vi "PBL2.vi"() -> ()   [LabVIEW 2017]
uses:
  C:/Users/mjoha/Documents/School/ELIC328/LabViewProject/FanCtrl/LabView Fan Controller.dll
  LabView Fan Controller.dll
panel:
  out "?":bool
  in  "COM Port":string
  in  "stop":bool
  in  "Temperature Settings":T1
  in  "?":enum32{"Output", "Settings", "Error Output"}(tab)
  out "Tempurate\nZone 2":dbl
  out "Tempurate\nZone 1":dbl
  out "Waveform Chart":T2(graph)
  in  "Zone 2":T3
  in  "Zone 1":T3
  out "error out":errorcluster
  # "Zone 1"
  # "Min"
  # "Max"
  # "Zone 2"
  # "Max"
  # "Min"
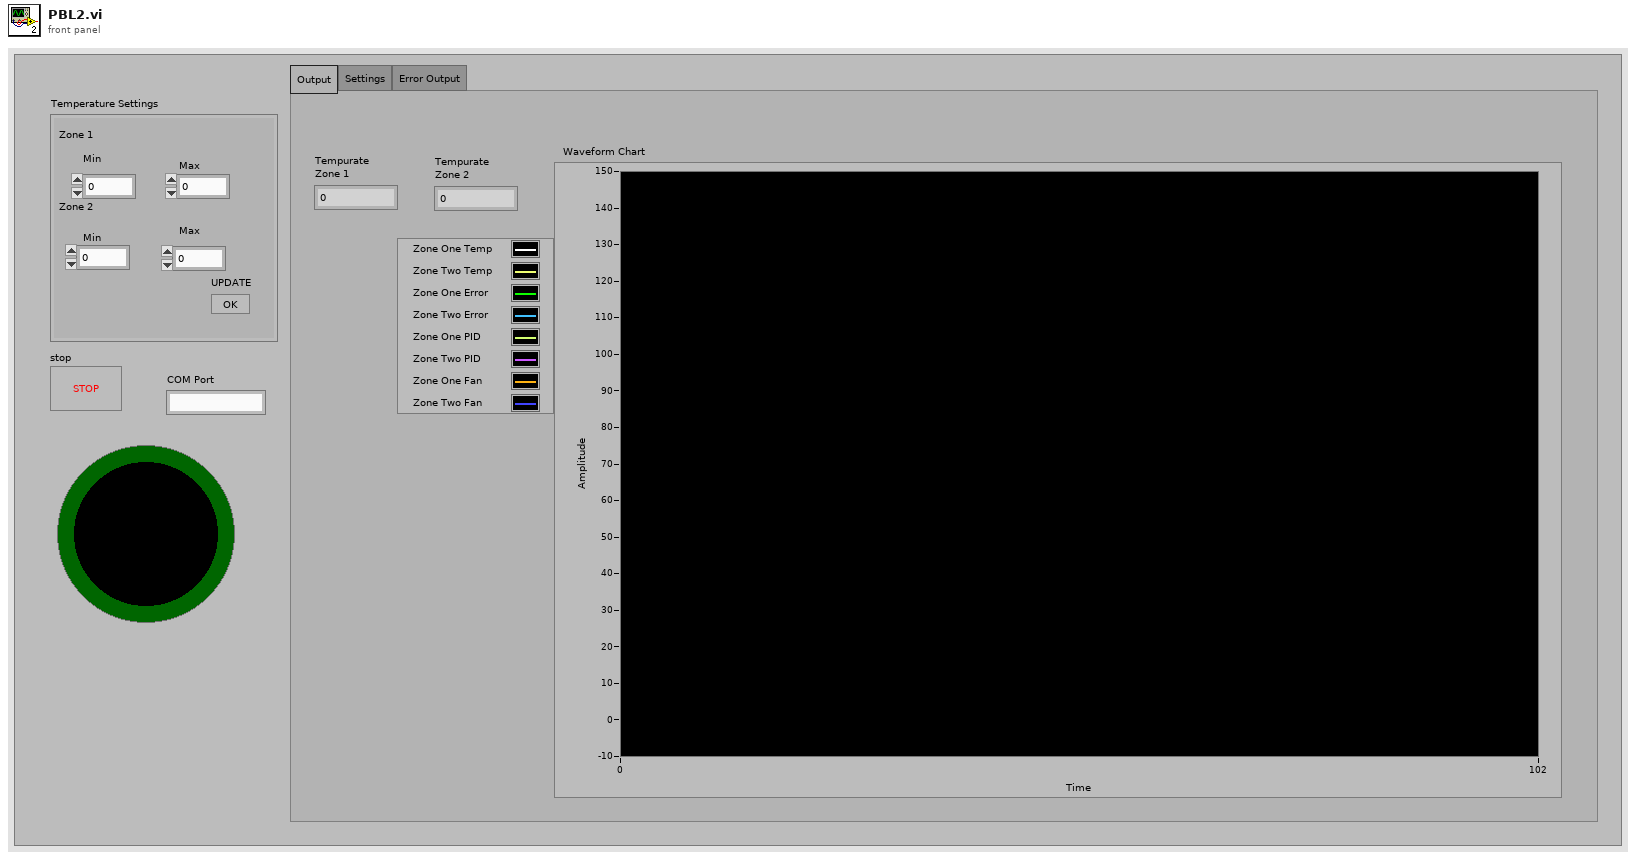
[diagram p1: front panel]
types:
  T1 = cluster{"Zone One Min Temp":dbl, "Zone One Max Temp":dbl, "Zone Two Min Temp":dbl, "Zone Two Max Temp":dbl, "UPDATE":bool}
  T2 = cluster{"ZoneTwoTemperature":dbl, "ZoneOneTemperature":dbl, "ZoneOneError":dbl, "ZoneTwoError":dbl, "ZoneOnePidRate":dbl, "ZoneTwoPidRate":dbl, "ZoneOneFanPwm":i32, "ZoneTwoFanPwm":i32}
  T3 = cluster{"KI":dbl, "KP":dbl, "KD":dbl, "Temp Samp":dbl, "Pid Samp":dbl}
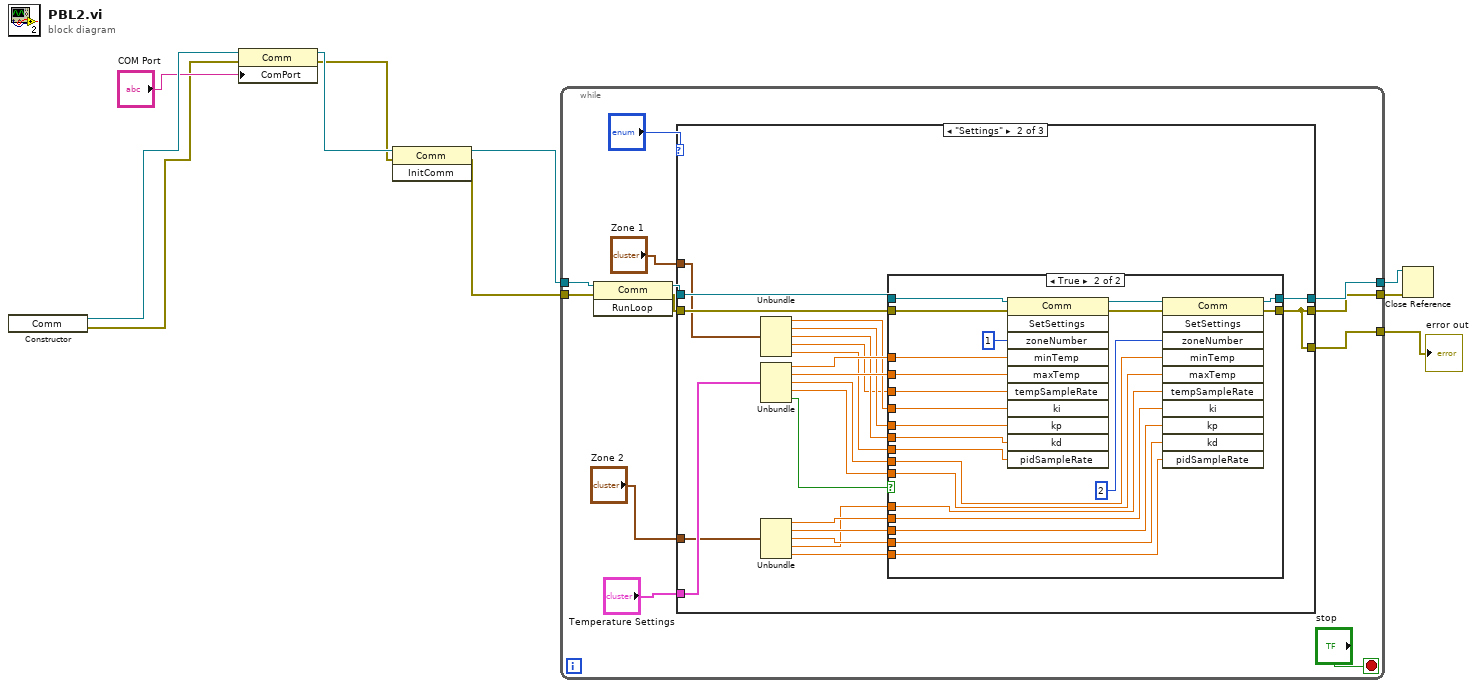
[diagram p0: block diagram]
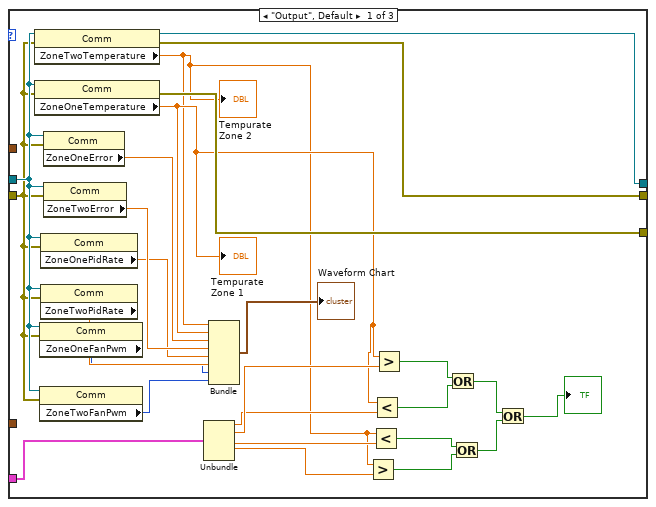
[diagram p2: hidden frame]
diagram:
  n1 = constructor class="Comm"() -> (reference out=w6:refnum<k24>, error out=w4:errorcluster)  [unwired: 3 in, 1 out]
  n2 = property class="Comm"(reference=w6, error in=w4, "ComPort"="COM Port") -> (reference out=w3:refnum<k24>, error out=w2:errorcluster)
  n3 = invoke class="Comm" method="InitComm"(reference=w3, error in=w2) -> (reference out=w8:refnum<k24>, error out=w7:errorcluster)  [unwired: 1 in, 1 out]
  n4 = while {
    tunnel: w8 -> [w19]
    tunnel: w7 -> [w18]
    tunnel: [w21] -> w10
    tunnel: [w20] -> w9
    tunnel: [w11] -> w1
    stop <- "stop" stop-if-true
    n5 = invoke class="Comm" method="RunLoop"(reference=w19, error in=w18) -> (reference out=w17:refnum<k24>, error out=w16:errorcluster)  [unwired: 1 in, 1 out]
    n6 = case shown="\"Settings\"" "?" {
      tunnel: w17 -> [w46 w69 w94]
      tunnel: w16 -> [w45 w68 w93]
      tunnel: [w48 w59 w94] -> w21
      tunnel: [w47 w50 w93] -> w20
      tunnel: "Temperature Settings" -> [w36 w70 _]
      tunnel: "Zone 1" -> [_ w65 _]
      tunnel: "Zone 2" -> [_ w58 _]
      tunnel: [w37 w50 w93] -> w11
      frame "Output", Default {
        n7 = property class="Comm"(reference=w46, error in=w45) -> (reference out=w48:refnum<k24>, error out=w47:errorcluster, "ZoneTwoTemperature"=w31:dbl)
        "Tempurate\nZone 2" <- w31
        n8 = property class="Comm"(reference=w46, error in=w45) -> (error out=w37:errorcluster, "ZoneOneTemperature"=w34:dbl)  [unwired: 1 out]
        "Tempurate\nZone 1" <- w34
        n9 = property class="Comm"(reference=w46, error in=w45) -> ("ZoneOneFanPwm"=w40:i32)  [unwired: 2 out]
        n10 = property class="Comm"(reference=w46, error in=w45) -> ("ZoneTwoFanPwm"=w39:i32)  [unwired: 2 out]
        n11 = property class="Comm"(reference=w46, error in=w45) -> ("ZoneOnePidRate"=w42:dbl)  [unwired: 2 out]
        n12 = property class="Comm"(reference=w46, error in=w45) -> ("ZoneTwoPidRate"=w41:dbl)  [unwired: 2 out]
        n13 = property class="Comm"(reference=w46, error in=w45) -> ("ZoneOneError"=w44:dbl)  [unwired: 2 out]
        n14 = property class="Comm"(reference=w46, error in=w45) -> ("ZoneTwoError"=w43:dbl)  [unwired: 2 out]
        n15 = Unbundle(w36) -> ("Zone One Min Temp"=w33:dbl, "Zone One Max Temp"=w35:dbl, "Zone Two Min Temp"=w32:dbl, "Zone Two Max Temp"=w30:dbl)  [unwired: 1 out]
        n16 = Bundle("ZoneTwoTemperature"=w31, "ZoneOneTemperature"=w34, "ZoneOneError"=w44, "ZoneTwoError"=w43, "ZoneOnePidRate"=w42, "ZoneTwoPidRate"=w41, "ZoneOneFanPwm"=w40, "ZoneTwoFanPwm"=w39) -> (→"Waveform Chart":T2)  [unwired: 1 in]
        n17 = Greater?(x=w31, y=w30) -> (0:w26:bool)
        n18 = Less?(x=w31, y=w32) -> (x < y?=w27:bool)
        n19 = Less?(x=w34, y=w33) -> (x < y?=w28:bool)
        n20 = Greater?(x=w34, y=w35) -> (0:w29:bool)
        n21 = Or(x=w29, y=w28) -> (x .or. y?=w25:bool)
        n22 = Or(x=w27, y=w26) -> (x .or. y?=w24:bool)
        n23 = Or(x=w25, y=w24) -> (x .or. y?=→"?":bool)
      }
      frame "Settings" {
        n24 = Unbundle(w65) -> ("KI"=w64:dbl, "KP"=w63:dbl, "KD"=w62:dbl, "Temp Samp"=w61:dbl, "Pid Samp"=w60:dbl)
        n25 = Unbundle(w70) -> ("Zone One Min Temp"=w67:dbl, "Zone One Max Temp"=w66:dbl, "Zone Two Min Temp"=w52:dbl, "Zone Two Max Temp"=w51:dbl, "UPDATE"=w49:bool)
        n26 = Unbundle(w58) -> ("KI"=w57:dbl, "KP"=w56:dbl, "KD"=w55:dbl, "Temp Samp"=w54:dbl, "Pid Samp"=w53:dbl)
        n27 = case shown="True" w49 {
          tunnel: w69 -> [_ w92]
          tunnel: w68 -> [_ w91]
          tunnel: [_ w79] -> w50
          tunnel: w67 -> [_ w89]
          tunnel: w66 -> [_ w88]
          tunnel: w64 -> [_ w87]
          tunnel: w63 -> [_ w86]
          tunnel: w62 -> [_ w85]
          tunnel: w61 -> [_ w84]
          tunnel: w60 -> [_ w83]
          tunnel: [_ w80] -> w59
          tunnel: w57 -> [_ w78]
          tunnel: w56 -> [_ w77]
          tunnel: w55 -> [_ w76]
          tunnel: w54 -> [_ w75]
          tunnel: w53 -> [_ w74]
          tunnel: w52 -> [_ w73]
          tunnel: w51 -> [_ w72]
          frame False {
          }
          frame True {
            n28 = invoke class="Comm" method="SetSettings"(reference=w92, error in=w91, "zoneNumber"=1, "minTemp"=w89, "maxTemp"=w88, "tempSampleRate"=w84, "ki"=w87, "kp"=w86, "kd"=w85, "pidSampleRate"=w83) -> (reference out=w82:refnum<k24>, error out=w81:errorcluster)  [unwired: 1 in, 9 out]
            n29 = invoke class="Comm" method="SetSettings"(reference=w82, error in=w81, "zoneNumber"=2, "minTemp"=w73, "maxTemp"=w72, "tempSampleRate"=w75, "ki"=w78, "kp"=w77, "kd"=w76, "pidSampleRate"=w74) -> (reference out=w80:refnum<k24>, error out=w79:errorcluster)  [unwired: 1 in, 9 out]
          }
        }
      }
      frame "Error Output" {
      }
    }
  }
  "error out" <- w1
  n30 = Close Reference(reference=w10, error in (no error)=w9) -> ()  [unwired: 1 out]
